vi "merge.vi"(8 "error in (no error)":errorcluster, 10 "update":refnum<class "GenericImagingMode.lvclass">, 11 "GenericScanMode in":refnum<class "GenericImagingMode.lvclass">) -> (0 "error out":errorcluster, 3 "GenericScanMode out":refnum<class "GenericImagingMode.lvclass">)   [LabVIEW 2010, in "GenericImagingMode.lvclass"]
uses:
  GenericImagingMode.lvclass
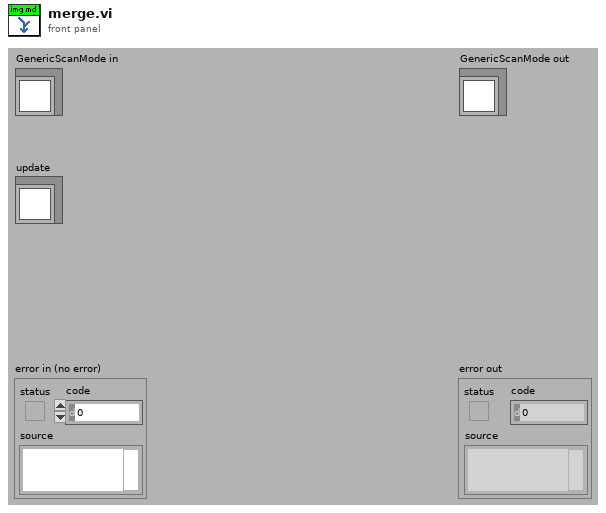
[diagram p1: front panel]
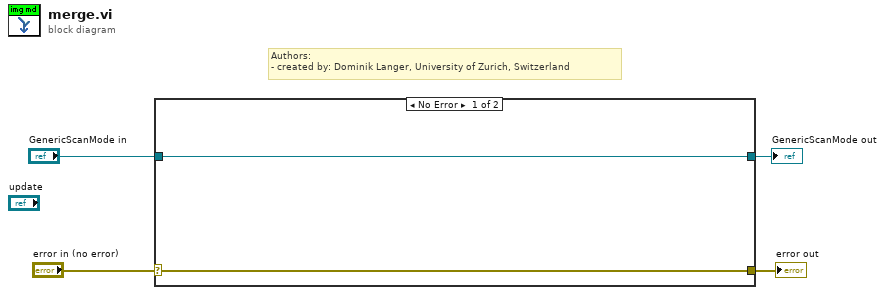
[diagram p0: block diagram]
diagram:
  # "Authors: \n- created by: Dominik Langer, University of Zurich, Switzerland"
  n1 = case shown="No Error" "error in (no error)" {
    selector: "error in (no error)" -> [w5 w8]
    tunnel: [w5 w8] -> w3
    tunnel: [w6 w7] -> w1
    tunnel: "GenericScanMode in" -> [w6 w7]
    frame No Error {
    }
    frame Error {
    }
  }
  "error out" <- w3
  "GenericScanMode out" <- w1
